vi "EIP_counter_UI.vi"(8 "error in (no error)":errorcluster, 9 "Boolean":bool, 10 "millisecond multiple":u32, 11 "VISA Refnum in":refnum<visa-resource-name>) -> (0 "error out":errorcluster, 2 "Dynamic Data Type":dynamicdata(waveform), 3 "Numeric":dbl)   [LabVIEW 2015]
uses:
  <vilib>/Utility/file.llb/Write Delimited Spreadsheet (string).vi
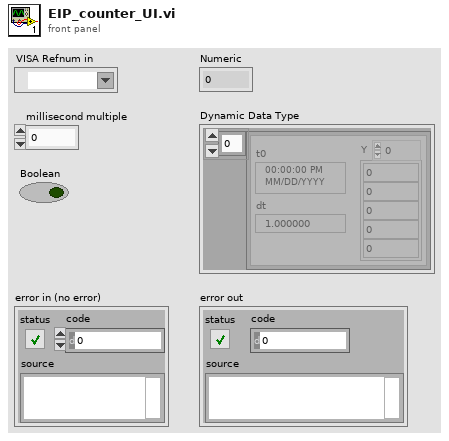
[diagram p1: front panel]
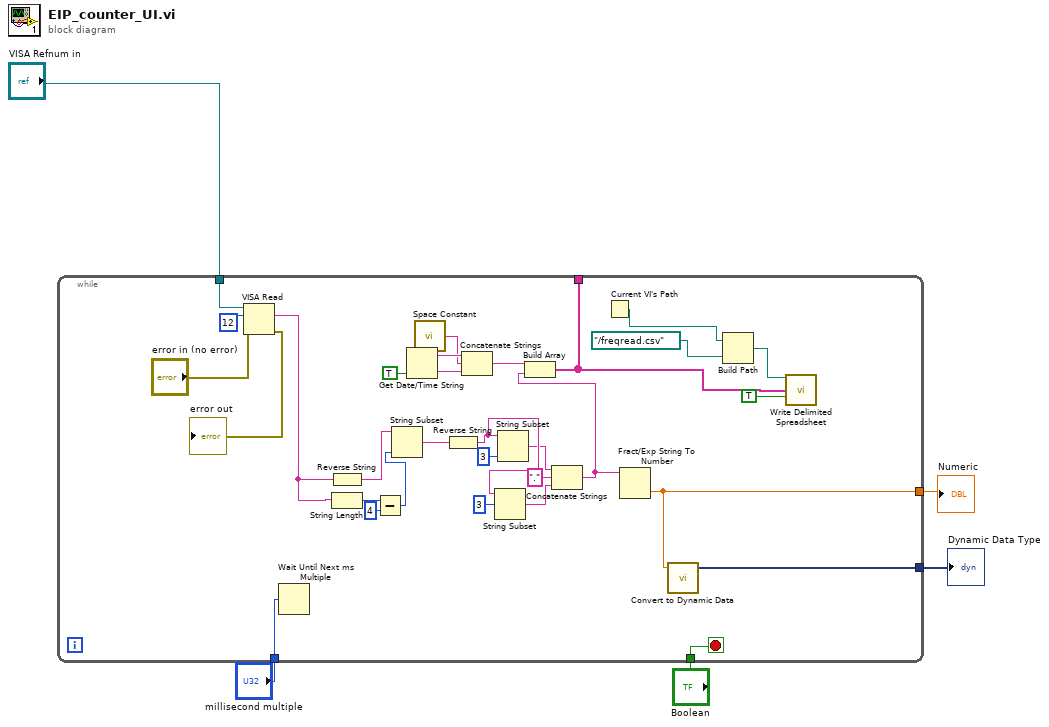
[diagram p0: block diagram]
diagram:
  n1 = while {
    tunnel: "VISA Refnum in" -> [w11]
    tunnel: [w10] -> w2
    tunnel: [w9] -> w3
    tunnel: [w8] -> _
    tunnel: "Boolean" -> [w7]
    tunnel: "millisecond multiple" -> [w6]
    stop <- w7 stop-if-true
    n2 = VISA Read(VISA resource name=w11, byte count=u32 12, error in (no error)="error in (no error)") -> (read buffer=w12:string, error out=→"error out":errorcluster)  [unwired: 2 out]
    n3 = Wait Until Next ms Multiple(millisecond multiple=w6) -> ()  [unwired: 1 out]
    n4 = Reverse String(1:w12) -> (0:w34:string)
    n5 = String Length(string=w12) -> (length=w36:i32)
    n6 = Subtract(x=w36, y=4) -> (x-y=w33:i32)
    n7 = String Subset(string=w34, length (rest)=w33) -> (substring=w32:string)  [unwired: 1 in]
    n8 = Get Date/Time String(want seconds? (F)=TRUE) -> (date string=w24:string, time string=w22:string)  [unwired: 2 in]
    n9 = call <vilib>:"Space Constant.vi"() -> ("String"=w23:string)
    n10 = Reverse String(1:w32) -> (0:w30:string)
    n11 = Concatenate Strings(w24, w23, w22) -> (w21:string)
    n12 = String Subset(string=w30, offset (0)=3) -> (substring=w28:string)  [unwired: 1 in]
    n13 = String Subset(string=w30, length (rest)=3 ("length (rest)")) -> (substring=w27:string)  [unwired: 1 in]
    n14 = Concatenate Strings(w27, "." ("string"), w28) -> (w20:string)
    n15 = Build Array(w21, w20) -> (w8:string[])
    n16 = Current VI's Path() -> (path=w17:path)
    n17 = Fract/Exp String To Number(string=w20) -> (number=w9:dbl)  [unwired: 3 in, 1 out]
    n18 = call "Convert to Dynamic Data"("Double"=w9) -> ("Dynamic Data Type"=w10:dynamicdata)  [unwired: 3 in]
    n19 = Build Path(base path=w17, name or relative path=path "../freqread.csv" ("base path")) -> (appended path=w18:path)
    n20 = call-poly <vilib>:"Write Delimited Spreadsheet.vi"("file path (dialog if empty)"=w18, "1D data"=w8, "append to file? (F)"=TRUE) -> ()  [unwired: 11 in, 2 out]
  }
  "Numeric" <- w3
  "Dynamic Data Type" <- w2
